vi "Delete TreePath DVR.vi"(8 "error in (no error)":errorcluster, 11 "TreePath DVR in":refnum<data-value>) -> (0 "error out":errorcluster, 3 "TreePath out":refnum<class "TreePath.lvclass">)   [LabVIEW 2013, in "MDSplus.lvlib" / "TreePath.lvclass"]
uses:
  <vilib>/MDSplus/Classes/Data_Class/TreeNode_Class/TreePath_Class/TreePath.lvclass
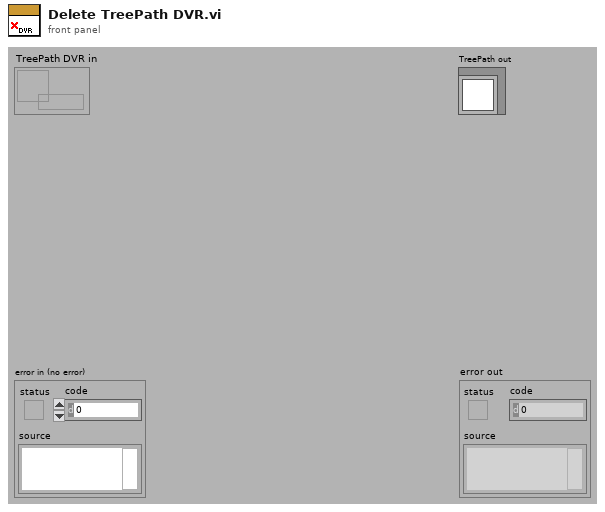
[diagram p1: front panel]
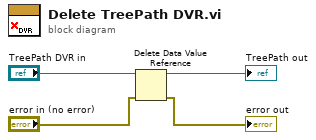
[diagram p0: block diagram]
diagram:
  n1 = Delete Data Value Reference(data value reference="TreePath DVR in", error in="error in (no error)") -> (data value=→"TreePath out":refnum<class "TreePath.lvclass">, error out=→"error out":errorcluster)
